vi "PI_SPA.vi"(8 "Value":u16, 9 "Register":string, 10 "Axis":string, 11 "Commandset in":string[](array[string])) -> (3 "Commandset out":string[](array[string]))   [LabVIEW 2011]
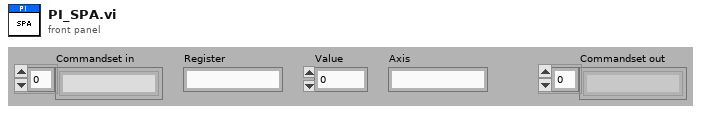
[diagram p1: front panel]
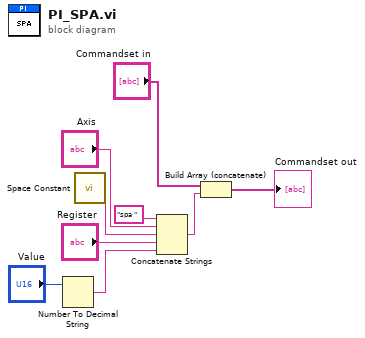
[diagram p0: block diagram]
diagram:
  n1 = Number To Decimal String(number="Value") -> (decimal integer string=w8:string)  [unwired: 1 out]
  n2 = call <vilib>:"Space Constant.vi"() -> ("String"=w6:string)
  n3 = Concatenate Strings("spa " ("new element/subarray"), "Axis", w6, "Register", w8) -> (w2:string)
  n4 = Build Array (concatenate)("Commandset in", w2) -> (→"Commandset out":string[])
